vi "Control-StatusText.vi"(1 "Parametros Actuales":T1, 2 "string":string) -> (0 "String":string)   [LabVIEW 2010]
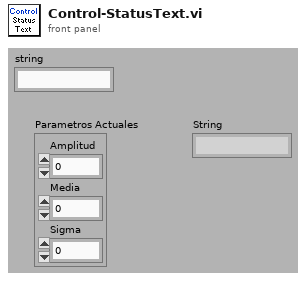
[diagram p1: front panel]
types:
  T1 = cluster{"Amplitud":dbl, "Media":dbl, "Sigma":dbl}
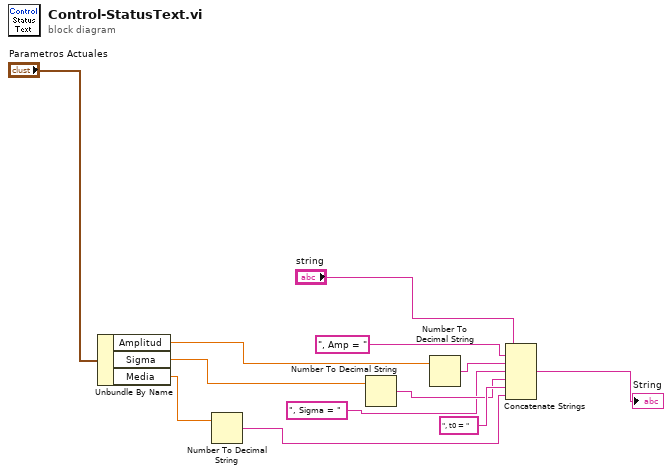
[diagram p0: block diagram]
diagram:
  n1 = Unbundle By Name("Parametros Actuales") -> ("Amplitud"=w10:dbl, "Sigma"=w11:dbl, "Media"=w12:dbl)
  n2 = Number To Decimal String(number=w12) -> (decimal integer string=w8:string)  [unwired: 1 in]
  n3 = Number To Decimal String(number=w11) -> (decimal integer string=w5:string)  [unwired: 1 in]
  n4 = Number To Decimal String(number=w10) -> (decimal integer string=w3:string)  [unwired: 1 in]
  n5 = Concatenate Strings("string", ", Amp = ", w3, ", Sigma = ", w5, ", t0 = " ("string"), w8) -> (→"String":string)
